vi "OP600ZP_CAN.vi"(5 "Tableau 3":string[][](array[string]), 9 "CAN_MESURES":cluster{string, string}) -> (1 "Tableau 2":string[][](array[string]), 4 "Tableau":bool[](array[boolean]))   [LabVIEW 2020]
uses:
  OP600ZP_VGConf.vi
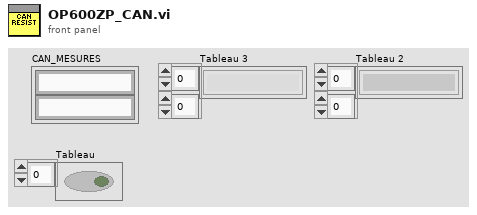
[diagram p1: front panel]
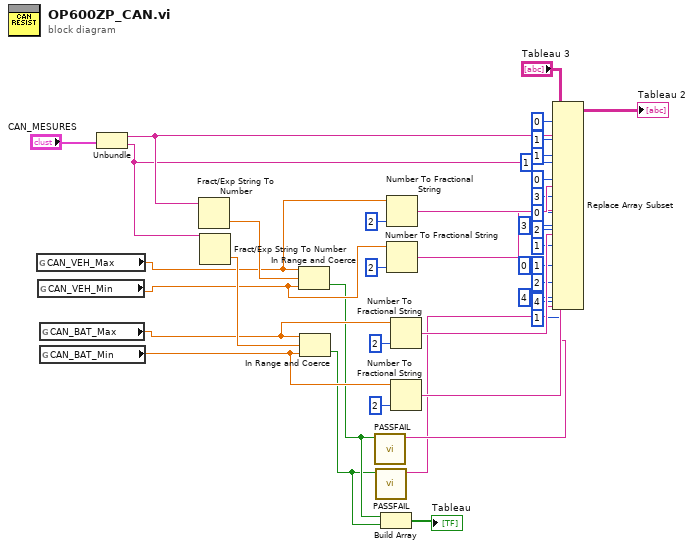
[diagram p0: block diagram]
diagram:
  n1 = global read "OP600ZP_VGConf.vi" "CAN_VEH_Max"() -> (w29:dbl)
  n2 = global read "OP600ZP_VGConf.vi" "CAN_VEH_Min"() -> (w28:dbl)
  n3 = global read "OP600ZP_VGConf.vi" "CAN_BAT_Max"() -> (w27:dbl)
  n4 = global read "OP600ZP_VGConf.vi" "CAN_BAT_Min"() -> (w26:dbl)
  n5 = Unbundle("CAN_MESURES") -> (w33:string, w32:string)
  n6 = Fract/Exp String To Number(string=w33) -> (number=w31:dbl)  [unwired: 3 in, 1 out]
  n7 = Fract/Exp String To Number(string=w32) -> (number=w30:dbl)  [unwired: 3 in, 1 out]
  n8 = In Range and Coerce(upper limit=w29, x=w31, lower limit=w28) -> (In Range?=w3:bool)  [unwired: 1 out]
  n9 = In Range and Coerce(upper limit=w27, x=w30, lower limit=w26) -> (In Range?=w2:bool)  [unwired: 1 out]
  n10 = call <vilib>:"PASSFAIL.vi"("E"=w3) -> ("S"=w9:string)  [unwired: 10 in]
  n11 = call <vilib>:"PASSFAIL.vi"("E"=w2) -> ("S"=w6:string)  [unwired: 10 in]
  n12 = Build Array(w3, w2) -> (→"Tableau":bool[])
  n13 = Number To Fractional String(number=w29, precision (6)=i16 2 ("précision (6)")) -> (F-format string=w21:string)  [unwired: 2 in]
  n14 = Number To Fractional String(number=w28, precision (6)=i16 2 ("précision (6)")) -> (F-format string=w18:string)  [unwired: 2 in]
  n15 = Number To Fractional String(number=w27, precision (6)=i16 2 ("précision (6)")) -> (F-format string=w15:string)  [unwired: 2 in]
  n16 = Number To Fractional String(number=w26, precision (6)=i16 2 ("précision (6)")) -> (F-format string=w12:string)  [unwired: 2 in]
  n17 = Replace Array Subset(array="Tableau 3", new element #1=w33, index (row) #1=0 ("indice (ligne)"), index (col) #1=1 ("indice désactivé (col)"), new element #2=w32, index (row) #2=1 ("indice (ligne)"), index (col) #2=1 ("indice désactivé (col)"), new element #3=w21, index (row) #3=0 ("indice (ligne)"), index (col) #3=3 ("indice désactivé (col)"), new element #4=w18, index (row) #4=0 ("indice (ligne)"), index (col) #4=2 ("indice désactivé (col)"), new element #5=w15, index (row) #5=1 ("indice (ligne)"), index (col) #5=3 ("indice désactivé (col)"), new element #6=w12, index (row) #6=1 ("indice (ligne)"), index (col) #6=2 ("indice désactivé (col)"), new element #7=w9, index (row) #7=0 ("indice (ligne)"), index (col) #7=4 ("indice désactivé (col)"), new element #8=w6, index (row) #8=1 ("indice (ligne)"), index (col) #8=4 ("indice désactivé (col)")) -> (→"Tableau 2":string[][])
